vi "Client - Initialize UI.vi"(8 "error in (no error)":errorcluster, 11 "Client - Data In":T1) -> (0 "error out":errorcluster, 3 "Client - Data Out":T1)   [LabVIEW 2024]
doc: "Initializes the client user interface."
uses:
  Controls/Client/Client - Data.ctl
  Shared/Message Queue/Client Message Queues.ctl
  Shared/Message Queue/Message Cluster.ctl
  Shared/Message Queue.lvlib
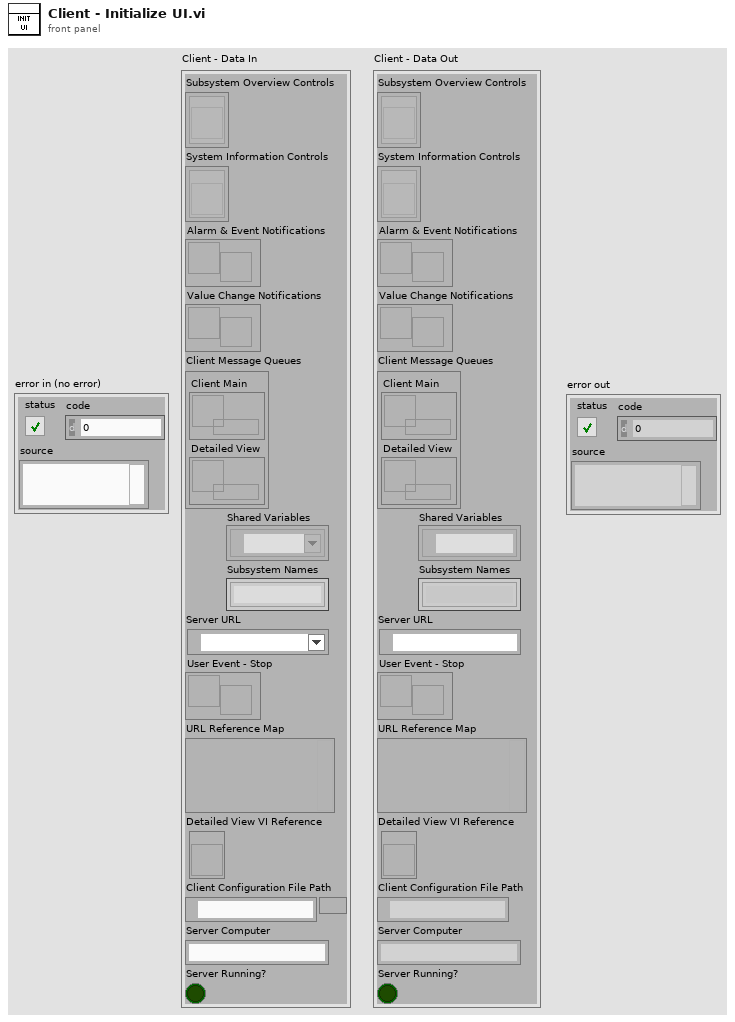
[diagram p1: front panel]
types:
  T1 = typedef "Client - Data.ctl" = cluster{"Subsystem Overview Controls":refnum<vi>[], "System Information Controls":refnum<vi>[], "Alarm & Event Notifications":refnum<user-event>, "Value Change Notifications":refnum<user-event>, "Client Message Queues":T2, "Shared Variables":refnum<k21>[], "Subsystem Names":string[], "Server URL":refnum<k21>, "User Event - Stop":refnum<user-event>, "URL Reference Map":variant, "Detailed View VI Reference":refnum<vi>, "Client Configuration File Path":path, "Server Computer":string, "Server Running?":bool}
  T2 = typedef "Message Queue.lvlib/Client Message Queues.ctl" = cluster{"Client Main":refnum<queue>, "Detailed View":refnum<queue>}
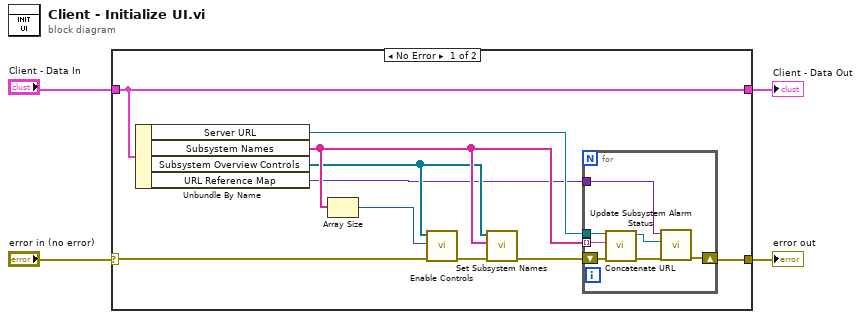
[diagram p0: block diagram]
diagram:
  n1 = case shown="No Error" "error in (no error)" {
    selector: "error in (no error)" -> [w5 w23]
    tunnel: [w7 w23] -> w3
    tunnel: "Client - Data In" -> [w12 w22]
    tunnel: [w12 w22] -> w1
    frame No Error {
      n2 = Unbundle By Name(w12) -> ("Server URL"=w10:refnum<k21>, "Subsystem Names"=w9:string[], "Subsystem Overview Controls"=w8:refnum<vi>[], "URL Reference Map"=w6:variant)
      n3 = Array Size(array=w9) -> (size(s)=w14:i32)
      n4 = call "Enable Controls.vi"("error in (no error)"=w5, "Number of Enabled Controls"=w14, "Controls"=w8) -> ("error out"=w13:errorcluster)  [unwired: 7 in, 1 out]
      n5 = call "Set Subsystem Names.vi"("error in (no error)"=w13, "Subsystem Names"=w9, "Subsystem Controls"=w8) -> ("error out"=w11:errorcluster)  [unwired: 7 in, 1 out]
      n6 = for {
        tunnel: w10 -> [w20]
        tunnel: w9 -> [w19] mode=indexing
        shift-right: [w17] -> w7
        shift-left: w11 -> [w21]
        tunnel: w6 -> [w16]
        n7 = call "Concatenate URL.vi"("error in (no error)"=w21, "Child Name"=w19, "Parent URL"=w20) -> ("error out"=w18:errorcluster, "Child URL"=w15:refnum<k21>)  [unwired: 7 in]
        n8 = call "Update Subsystem Alarm Status.vi"("error in (no error)"=w18, "Subsystem URL"=w15, "Reference URL Map In"=w16) -> ("error out"=w17:errorcluster)  [unwired: 7 in, 1 out]
      }
    }
    frame Error {
    }
  }
  "error out" <- w3
  "Client - Data Out" <- w1
